vi "LidarTester.vi"() -> ()   [LabVIEW 2024]
uses:
  e33ea129-5426-40bd-9da2-e127971607b1.vi
  <vilib>/Instr/_visa.llb/VISA Configure Serial Port (Instr).vi
panel:
  in  "Tab Control":enum32{"Lidar", "Buffer"}(tab)
  out "LiDAR_ROI":cluster{i32[], i32[]}(graph)
  in  "COM4 2":refnum<visa-resource-name>="COM3" caption="LiDAR_Com."
  in  "격자크기":dbl=20.0
  in  "Stop":bool
  out "Loop Time":u32=102
  out "read buffer":string
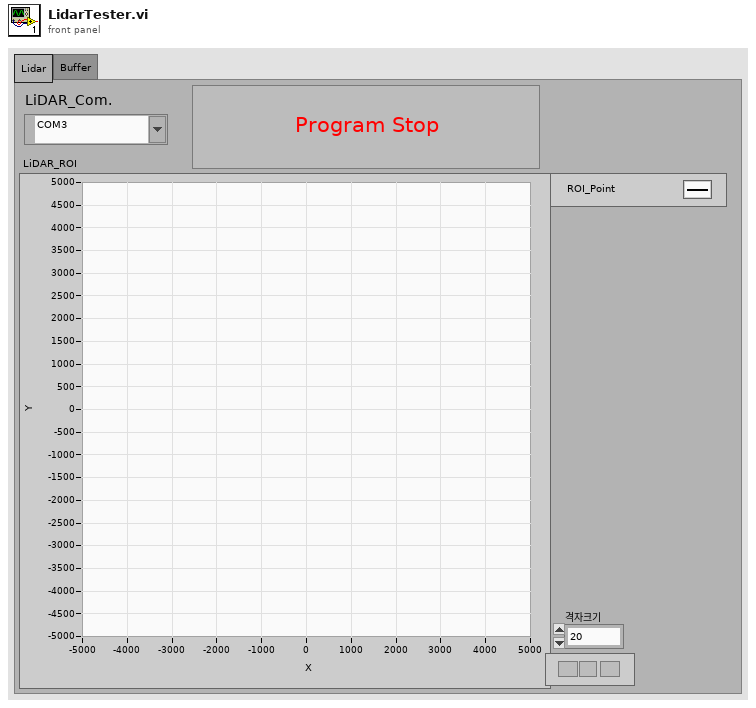
[diagram p1: front panel]
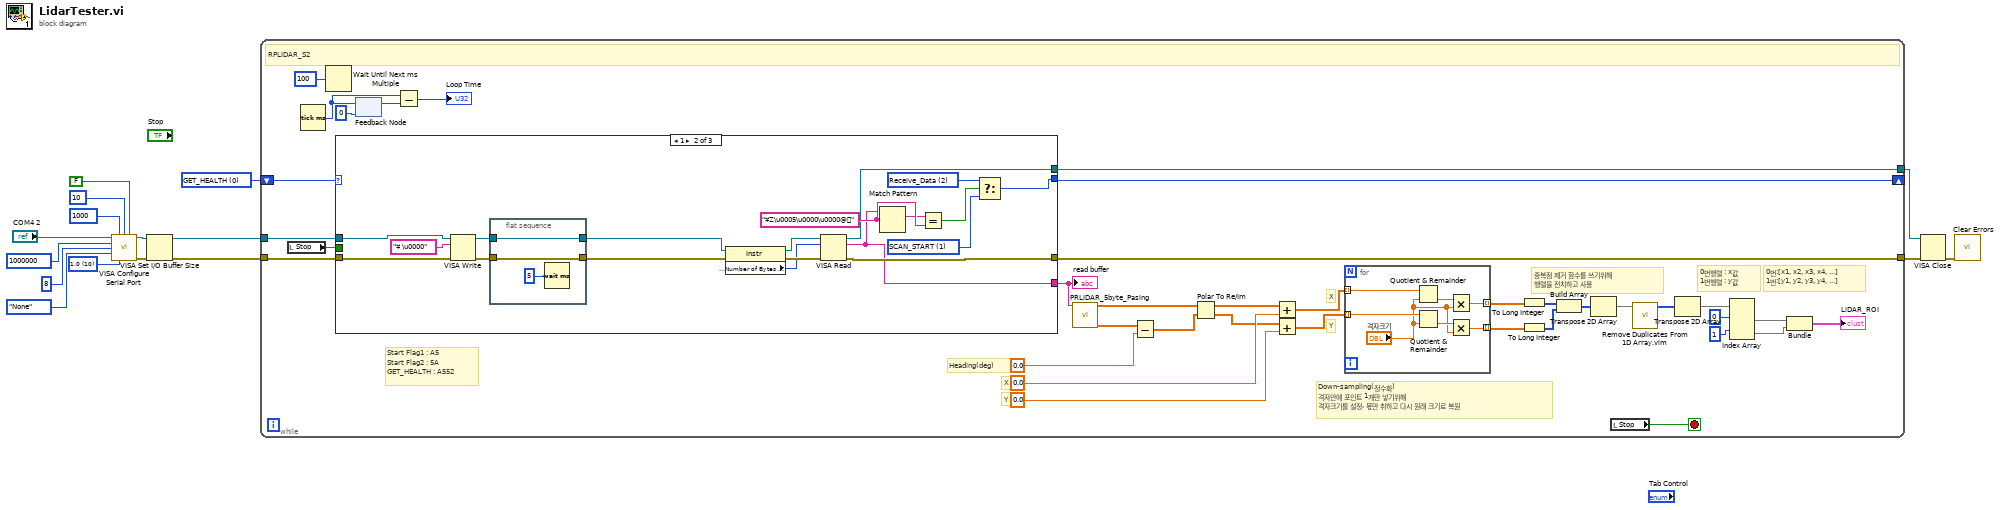
[diagram p0: block diagram]
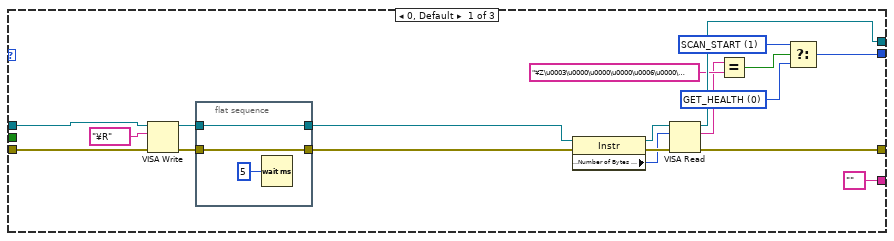
[diagram p2: hidden frame]
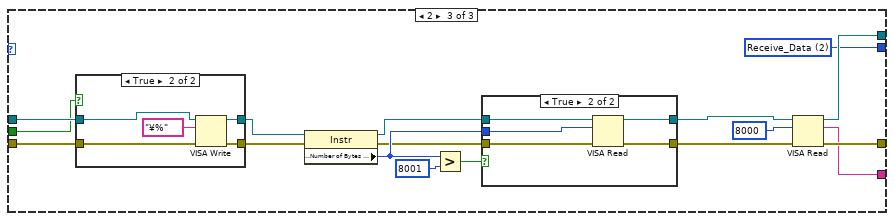
[diagram p3: hidden frame]
diagram:
  w1 = u16 10 items=["1.0"=10, "1.5"=15, "2.0"=20] ("stop bits (10: 1 bit)")
  w3 = u16 0 items=["GET_HEALTH", "SCAN_START", "Receive_Data"]
  n1 = call-poly "VISA Configure Serial Port"("VISA resource name"="COM4 2", "timeout (10sec)"=u32 1000, "termination char\n(0xA = '\\n' = LF)"=u8 10 ("termination char\n(0xA = '\\n' = LF)"), "Enable Termination\nChar (T)"=FALSE ("Enable Termination\nChar (T)"), "baud rate (9600)"=u32 1000000, "data bits (8)"=u16 8, "parity (0:none)"=enum16{"None", "Odd", "Even", "Mark", "Space"}."None", "stop bits (10: 1 bit)"=w1) -> ("VISA resource name out"=w11:refnum<visa-resource-name>, "error out"=w10:errorcluster)  [unwired: 6 in]
  n2 = VISA Set I/O Buffer Size(VISA resource name=w11, error in (no error)=w10) -> (VISA resource name out=w5:refnum<visa-resource-name>, error out=w4:errorcluster)  [unwired: 2 in]
  n3 = while {
    tunnel: [w43] -> w15
    tunnel: [w44] -> w14
    tunnel: w5 -> [w52]
    tunnel: w4 -> [w51]
    shift-right: [w50] -> _
    shift-left: w3 -> [w53]
    stop <- w30 stop-if-true
    # "Y"
    # "X"
    # "Heading(deg)"
    # "Start Flag1 : A5\nStart Flag2 : 5A \nGET_HEALTH : A552"
    # "0번:[x1, x2, x3, x4, ...]\n1번:[y1, y2, y3, y4, ...]"
    # "0번행렬 : x값\n1번행렬 : y값"
    # "중복점 제거 함수를 쓰기위해\n행렬을 전치하고 사용"
    # "Down-sampling(정수화)\n격자안에 포인트 1개만 넣기위해\n격자크기를 설정, 몫만 취하고 다시 원래 크기로 복원"
    # "Y"
    # "X"
    # "RPLIDAR_S2"
    n4 = local read "Stop"() -> (w49:bool)
    n5 = Tick Count (ms)() -> (millisecond timer value=w48:u32)
    n6 = Wait Until Next ms Multiple(millisecond multiple=u32 100 ("ms 배수")) -> ()  [unwired: 1 out]
    n7 = case shown="1" w53 {
      tunnel: w52 -> [w78 w96 w119]
      tunnel: w51 -> [w77 w95 w118]
      tunnel: [w79 w92 w105] -> w50
      tunnel: [w68 w93 w121] -> w44
      tunnel: [w67 w94 w120] -> w43
      tunnel: w49 -> [_ _ w117]
      tunnel: ["" ("read buffer") w90 w116] -> w31
      frame 0, Default {
        w61 = u16 0 items=["GET_HEALTH", "SCAN_START", "Receive_Data"]
        w62 = u16 1 items=["GET_HEALTH", "SCAN_START", "Receive_Data"]
        n8 = VISA Write(VISA resource name=w78, write buffer="¥R", error in (no error)=w77) -> (VISA resource name out=w72:refnum<visa-resource-name>, error out=w71:errorcluster)  [unwired: 1 out]
        n9 = flat-sequence {
          tunnel: w72 -> [w81]
          tunnel: w71 -> [w80]
          tunnel: [w81] -> w70
          tunnel: [w80] -> w69
          frame #0 {
            n10 = Wait (ms)(milliseconds to wait=u32 5 ("대기 시간 (ms)")) -> ()  [unwired: 1 out]
          }
        }
        n11 = property class="Instr"(reference=w70, error in=w69) -> (reference out=w75:refnum<visa-resource-name>, error out=w74:errorcluster, "Serial Settings:Number of Bytes at Serial Port"=w73:u32)
        n12 = VISA Read(VISA resource name=w75, byte count=w73, error in (no error)=w74) -> (VISA resource name out=w67:refnum<visa-resource-name>, read buffer=w64:string, error out=w68:errorcluster)  [unwired: 1 out]
        n13 = Equal?(x=w64, y="¥Z\u0003\u0000\u0000\u0000\u0006\u0000\u0000\u0000") -> (x = y?=w65:bool)
        n14 = Select(t=w62, s=w65, f=w61) -> (s? t:f=w79:u16)
      }
      frame 1 {
        w83 = u16 2 items=["GET_HEALTH", "SCAN_START", "Receive_Data"]
        w84 = u16 1 items=["GET_HEALTH", "SCAN_START", "Receive_Data"]
        w97 = "¥Z\u0005\u0000\u0000@"
        n15 = VISA Write(VISA resource name=w96, write buffer="¥ \u0000", error in (no error)=w95) -> (VISA resource name out=w99:refnum<visa-resource-name>, error out=w100:errorcluster)  [unwired: 1 out]
        n16 = flat-sequence {
          tunnel: w99 -> [w103]
          tunnel: w100 -> [w102]
          tunnel: [w103] -> w86
          tunnel: [w102] -> w85
          frame #0 {
            n17 = Wait (ms)(milliseconds to wait=u32 5 ("대기 시간 (ms)")) -> ()  [unwired: 1 out]
          }
        }
        n18 = property class="Instr"(reference=w86, error in=w85) -> (reference out=w89:refnum<visa-resource-name>, error out=w88:errorcluster, "Serial Settings:Number of Bytes at Serial Port"=w87:u32)
        n19 = VISA Read(VISA resource name=w89, byte count=w87, error in (no error)=w88) -> (VISA resource name out=w94:refnum<visa-resource-name>, read buffer=w90:string, error out=w93:errorcluster)  [unwired: 1 out]
        n20 = Match Pattern(string=w90, regular expression=w97) -> (match substring=w91:string)  [unwired: 1 in, 3 out]
        n21 = Equal?(x=w91, y=w97) -> (x = y?=w101:bool)
        n22 = Select(t=w83, s=w101, f=w84) -> (s? t:f=w92:u16)
      }
      frame 2 {
        w105 = u16 2 items=["GET_HEALTH", "SCAN_START", "Receive_Data"]
        n23 = case shown="True" w117 {
          tunnel: w119 -> [w130 w134]
          tunnel: w118 -> [w129 w133]
          tunnel: [w130 w132] -> w115
          tunnel: [w129 w131] -> w114
          frame False {
          }
          frame True {
            n24 = VISA Write(VISA resource name=w134, write buffer="¥%", error in (no error)=w133) -> (VISA resource name out=w132:refnum<visa-resource-name>, error out=w131:errorcluster)  [unwired: 1 out]
          }
        }
        n25 = property class="Instr"(reference=w115, error in=w114) -> (reference out=w110:refnum<visa-resource-name>, error out=w109:errorcluster, "Serial Settings:Number of Bytes at Serial Port"=w111:u32)
        n26 = Greater?(x=w111, y=u32 8001) -> (0:w113:bool)
        n27 = case shown="True" w113 {
          tunnel: w110 -> [w123 w128]
          tunnel: w111 -> [_ w127]
          tunnel: w109 -> [w122 w126]
          tunnel: [w123 w125] -> w108
          tunnel: [w122 w124] -> w107
          frame False {
          }
          frame True {
            n28 = VISA Read(VISA resource name=w128, byte count=w127, error in (no error)=w126) -> (VISA resource name out=w125:refnum<visa-resource-name>, error out=w124:errorcluster)  [unwired: 2 out]
          }
        }
        n29 = VISA Read(VISA resource name=w108, byte count=u32 8000, error in (no error)=w107) -> (VISA resource name out=w120:refnum<visa-resource-name>, read buffer=w116:string, error out=w121:errorcluster)  [unwired: 1 out]
      }
    }
    "read buffer" <- w31
    n30 = feedback #1(u32 0 ("millisecond timer value")) -> (w47:u32)
    n31 = feedback-in #1(w48) -> ()
    n32 = Subtract(x=w48, y=w47) -> (x-y=→"Loop Time":u32)
    n33 = call "PRLIDAR_5byte_Pasing.vi"("RPLIDAR_Data"=w31) -> ("Theta(deg)"=w25:dbl[], "Distance(mm)"=w26:dbl[])  [unwired: 9 in]
    n34 = Subtract(x=w25, y=0.0) -> (x-y=w23:dbl[])
    n35 = Polar To Re/Im(2:w23, 3:w26) -> (0:w19:dbl[], 1:w20:dbl[])
    n36 = Add(x=w20, y=0.0) -> (x+y=w18:dbl[])
    n37 = Add(x=w19, y=0.0) -> (x+y=w17:dbl[])
    n38 = for {
      tunnel: w18 -> [w60] mode=indexing
      tunnel: w17 -> [w59] mode=indexing
      tunnel: [w56] -> w41 mode=indexing
      tunnel: [w55] -> w42 mode=indexing
      n39 = Quotient & Remainder(x=w60, y="격자크기") -> (floor(x/y)=w58:dbl)  [unwired: 1 out]
      n40 = Quotient & Remainder(x=w59, y="격자크기") -> (floor(x/y)=w57:dbl)  [unwired: 1 out]
      n41 = Multiply(x=w58, y="격자크기") -> (x*y=w56:dbl)
      n42 = Multiply(x=w57, y="격자크기") -> (x*y=w55:dbl)
    }
    n43 = To Long Integer(number=w41) -> (32bit integer=w35:i32[])
    n44 = To Long Integer(number=w42) -> (32bit integer=w34:i32[])
    n45 = Build Array(w35, w34) -> (w37:i32[][])
    n46 = Transpose 2D Array(2D array=w37) -> (transposed array=w32:i32[][])
    n47 = local read "Stop"() -> (w30:bool)
    n48 = call "Remove Duplicates From 1D Array.vim"("array"=w32) -> ("array with duplicates removed"=w33:i32[][])  [unwired: 10 in]
    n49 = Transpose 2D Array(2D array=w33) -> (transposed array=w38:i32[][])
    n50 = Index Array(array=w38, index (row) #1=0 ("index (row)"), index (row) #2=1 ("index (row)")) -> (element #1=w29:i32[], element #2=w28:i32[])  [unwired: 2 in]
    n51 = Bundle(w29, w28) -> (→"LiDAR_ROI":cluster{i32[], i32[]})  [unwired: 1 in]
  }
  n52 = VISA Close(VISA resource name=w15, error in (no error)=w14) -> (error out=w16:errorcluster)
  n53 = call <vilib>:"Clear Errors.vi"("error in (no error)"=w16) -> ()  [unwired: 5 in, 2 out]
